vi "Dequeue Incoming Data.vi"(8 "error in":errorcluster, 11 "server in":refnum<class "RT FlexRIO Server TCP.lvclass">) -> (0 "error out":errorcluster, 2 "string out":string, 3 "server out":refnum<class "RT FlexRIO Server TCP.lvclass">)   [LabVIEW 2017, in "RT FlexRIO Server TCP.lvclass"]
uses:
  RT FlexRIO Server TCP.lvclass
  Properties/IncomingQueue_GET.vi
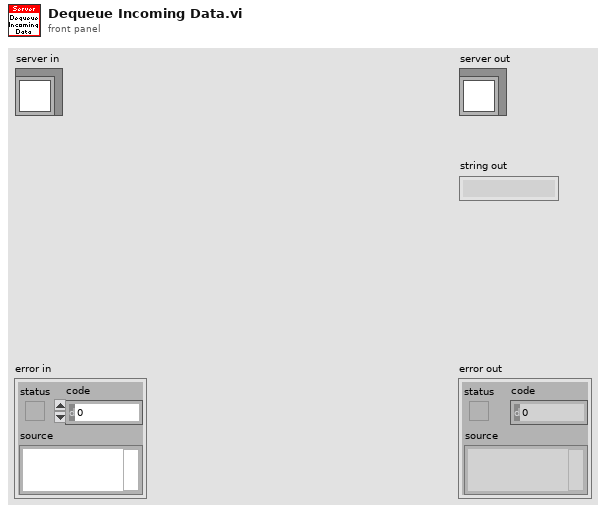
[diagram p1: front panel]
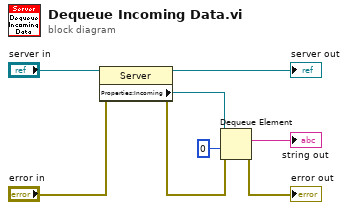
[diagram p0: block diagram]
diagram:
  n1 = property class="Server"(reference="server in", error in="error in") -> (reference out=→"server out":refnum<class "RT FlexRIO Server TCP.lvclass">, error out=w2:errorcluster, "Properties:Incoming"=w6:refnum<queue>)
  n2 = Dequeue Element(queue=w6, timeout in ms (-1)=0, error in (no error)=w2) -> (element=→"string out":string, error out=→"error out":errorcluster)  [unwired: 2 out]
